vi "PlayAlarm - Copy.vi"(8 "wavefilename":string, 11 "alertvolume":u16) -> ()   [LabVIEW 2011]
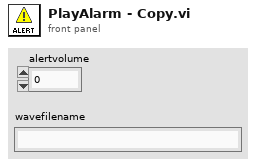
[diagram p1: front panel]
types:
  T1 = typedef "Sound Format.ctl" = cluster{"sound quality":enum16{"mono", "stereo"}, "rate":enum16{"11025", "22050", "44100", "8000"}, "bits per sample":enum16{"8 bit", "16 bit"}}
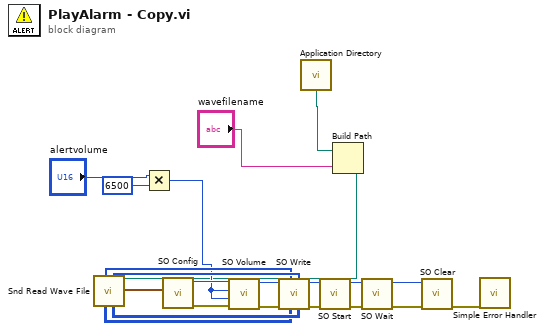
[diagram p0: block diagram]
diagram:
  n1 = Multiply(x="alertvolume", y=u16 6500) -> (x*y=w6:u16)
  n2 = call <vilib>:"Application Directory.vi"() -> ("Application Directory"=w2:path)
  n3 = Build Path(base path=w2, name or relative path="wavefilename") -> (appended path=w3:path)
  n4 = call <vilib>:"Snd Read Wave File.vi"("wave file path"=w3) -> ("sound format"=w20:T1, "stereo 16-bit"=w13:i16[][], "mono 16-bit"=w15:i16[], "stereo 8-bit"=w12:u8[][], "mono 8-bit"=w14:u8[])  [unwired: 4 in, 2 out]
  n5 = call <vilib>:"SO Config.vi"("sound format"=w20) -> ("error out"=w16:errorcluster, "task ID out"=w17:u32)  [unwired: 9 in]
  n6 = call <vilib>:"SO Volume.vi"("error in (no error)"=w16, "right channel"=w6, "left channel"=w6, "task ID in"=w17) -> ("error out"=w19:errorcluster, "task ID out"=w18:u32)  [unwired: 6 in]
  n7 = call <vilib>:"SO Write.vi"("stereo 16-bit"=w13, "mono 16-bit"=w15, "stereo 8-bit"=w12, "mono 8-bit"=w14, "error in (no error)"=w19, "task ID in"=w18) -> ("error out"=w10:errorcluster, "task ID out"=w11:u32)  [unwired: 4 in]
  n8 = call <vilib>:"SO Start.vi"("error in (no error)"=w10, "task ID in"=w11) -> ("error out"=w9:errorcluster, "task ID out"=w8:u32)  [unwired: 8 in]
  n9 = call <vilib>:"SO Wait.vi"("error in (no error)"=w9, "task ID in"=w8) -> ("error out"=w22:errorcluster, "task ID out"=w21:u32)  [unwired: 8 in]
  n10 = call <vilib>:"SO Clear.vi"("error in (no error)"=w22, "task ID in"=w21) -> ("error out"=w7:errorcluster)  [unwired: 9 in]
  n11 = call <vilib>:"Simple Error Handler.vi"("error in (no error)"=w7) -> ()  [unwired: 4 in, 5 out]
